vi "dfd_MRate_Calculate Filter Gain.vi"(9 "scale type":T3=enum."Time Domain 1-Norm", 10 "scale by Power of 2?":bool, 11 "multirate filter in":T1={"mMRate_Structure"=enum."CIC", "mMRate_Mode"=0, "mMRate_Factor"=0, "mMRate_FIRParams"={"mMRate_FIR_H"=[], "mMRate_FIR_IsNyquist?"=FALSE, "mMRate_FIR_IsSymmetric?"=FALSE}, "mMRate_CICParams"={"mMRate_CIC_#Stage"=0, "mMRate_CIC_Lag"=0, "mMRate_CIC_Type"=enum."Lowpass"}, "mMRate_Order"=0, "mMRate_Version"="", "mMRate_Comments"="", "mMRate_RationalFactor"={"mMRate_L"=-1, "mMRate_M"=-1}, "mMRate_Fs"=0.0, "mMRate_Quantized?"=FALSE, "mMRate_QFilterGain"=1.0, "mMRate_CoefWl"=16, "mMRate_Scaling"={"mMRate_ScaleByPowerOf2?"=FALSE, "mMRate_ScaleType"=enum."Time Domain 1-Norm"}, "mMRate_InputWl"=0, "mMRate_OutputWl"=0, "mMRate_OutputMode"=enum."Nearest", "mMRate_MultMode"=enum."Truncated", "mMRate_BitPruning"=FALSE, "mMRate_GainWl"=16, "mMRate_OutputFwl"=0, "mMRate_SumIwl"=0, "mMRate_InputIwl "=16, "mMRate_SumWl"=32, "mMRate_CoefIwl"=0} {"mMRate_SumWl" min=1 max=32 step=1; "mMRate_InputIwl" min=1 max=32 step=1; "mMRate_GainWl" min=1 max=32 step=1; "mMRate_OutputWl" min=1 max=32 step=1; "mMRate_InputWl" min=1 max=32 step=1; "mMRate_CoefWl" min=1 max=32 step=1; "mMRate_Mode" items=["Default"=-1, "No Rate Change"=0, "Interpolation"=1, "Decimation"=2, "Interpolated"=3, "Rational"=4]}) -> (1 "sum iwl":i16, 2 "scaled gain":dbl, 3 "dup multirate filter":T1={"mMRate_Structure"=enum."CIC", "mMRate_Mode"=0, "mMRate_Factor"=0, "mMRate_FIRParams"={"mMRate_FIR_H"=[], "mMRate_FIR_IsNyquist?"=FALSE, "mMRate_FIR_IsSymmetric?"=FALSE}, "mMRate_CICParams"={"mMRate_CIC_#Stage"=0, "mMRate_CIC_Lag"=0, "mMRate_CIC_Type"=enum."Lowpass"}, "mMRate_Order"=0, "mMRate_Version"="", "mMRate_Comments"="", "mMRate_RationalFactor"={"mMRate_L"=-1, "mMRate_M"=-1}, "mMRate_Fs"=0.0, "mMRate_Quantized?"=FALSE, "mMRate_QFilterGain"=1.0, "mMRate_CoefWl"=16, "mMRate_Scaling"={"mMRate_ScaleByPowerOf2?"=FALSE, "mMRate_ScaleType"=enum."Time Domain 1-Norm"}, "mMRate_InputWl"=0, "mMRate_OutputWl"=0, "mMRate_OutputMode"=enum."Nearest", "mMRate_MultMode"=enum."Truncated", "mMRate_BitPruning"=FALSE, "mMRate_GainWl"=16, "mMRate_OutputFwl"=0, "mMRate_SumIwl"=0, "mMRate_InputIwl "=16, "mMRate_SumWl"=32, "mMRate_CoefIwl"=0} {"mMRate_SumWl" min=1 max=32 step=1; "mMRate_InputIwl" min=1 max=32 step=1; "mMRate_GainWl" min=1 max=32 step=1; "mMRate_OutputWl" min=1 max=32 step=1; "mMRate_InputWl" min=1 max=32 step=1; "mMRate_CoefWl" min=1 max=32 step=1; "mMRate_Mode" items=["Default"=-1, "No Rate Change"=0, "Interpolation"=1, "Decimation"=2, "Interpolated"=3, "Rational"=4]})   [LabVIEW 2017, in "NI_DigFilter_FXP.lvlib"]
uses:
  <vilib>/addons/Digital Filter Design/NI_DigFilter_FXP.lvlib
  <vilib>/addons/Digital Filter Design/_Objects.llb/DFD Coef Norm Type.ctl
  <vilib>/addons/Digital Filter Design/_Objects.llb/DFD Multirate Filter Obj.ctl
  <vilib>/addons/Digital Filter Design/_Objects.llb/DFD Multirate Mode.ctl
  <vilib>/addons/Digital Filter Design/_Objects.llb/DFD Round-off Mode.ctl
  <vilib>/addons/Digital Filter Design/_Objects.llb/DFD FXP MRate Multiply Mode.ctl
  <vilib>/addons/Digital Filter Design/NI_DigFilterLicensed.lvlib
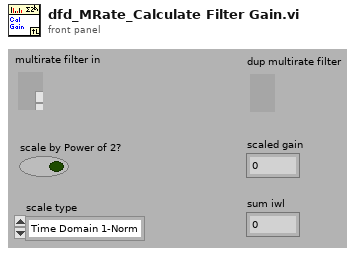
[diagram p1: front panel]
types:
  T1 = typedef "NI_DigFilterLicensed.lvlib/DFD Multirate Filter Obj.ctl" = cluster{"mMRate_Structure":enum16{"CIC", "FIR", "IIR", "Lattice"}, "mMRate_Mode":T2, "mMRate_Factor":i32, "mMRate_FIRParams":cluster{"mMRate_FIR_H":dbl[], "mMRate_FIR_IsNyquist?":bool, "mMRate_FIR_IsSymmetric?":bool}, "mMRate_CICParams":cluster{"mMRate_CIC_#Stage":i32, "mMRate_CIC_Lag":i32, "mMRate_CIC_Type":enum16{"Lowpass", "Highpass"}}, "mMRate_Order":i32, "mMRate_Version":string, "mMRate_Comments":string, "mMRate_RationalFactor":cluster{"mMRate_L":i32, "mMRate_M":i32}, "mMRate_Fs":dbl, "mMRate_Quantized?":bool, "mMRate_QFilterGain":dbl, "mMRate_CoefWl":i16, "mMRate_Scaling":cluster{"mMRate_ScaleByPowerOf2?":bool, "mMRate_ScaleType":T3}, "mMRate_InputWl":i16, "mMRate_OutputWl":i16, "mMRate_OutputMode":T4, "mMRate_MultMode":T5, "mMRate_BitPruning":bool, "mMRate_GainWl":i16, "mMRate_OutputFwl":i16, "mMRate_SumIwl":i16, "mMRate_InputIwl ":i16, "mMRate_SumWl":i16, "mMRate_CoefIwl":i16}
  T2 = typedef "NI_DigFilterLicensed.lvlib/DFD Multirate Mode.ctl" = i16
  T3 = typedef "NI_DigFilterLicensed.lvlib/DFD Coef Norm Type.ctl" = enum16{"No Norm", "Time Domain 1-Norm", "Time Domain 2-Norm", "Time Domain Inf-Norm"}
  T4 = typedef "NI_DigFilterLicensed.lvlib/DFD Round-off Mode.ctl" = enum16{"Nearest", "Truncation"}
  T5 = typedef "NI_DigFilterLicensed.lvlib/DFD FXP MRate Multiply Mode.ctl" = enum16{"Truncated", "Full"}
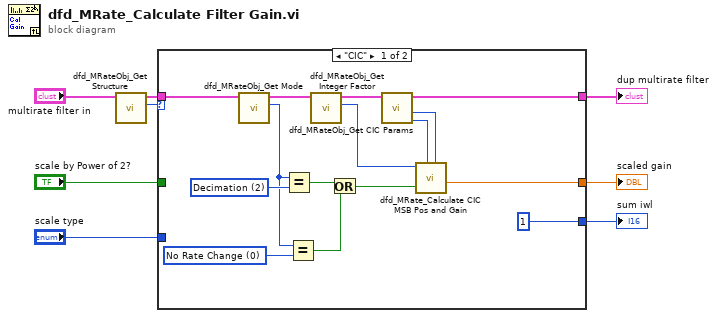
[diagram p0: block diagram]
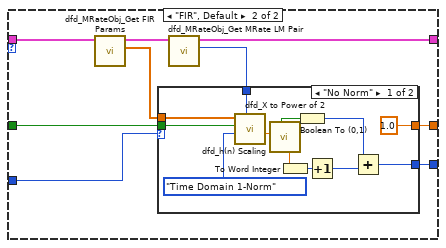
[diagram p2: hidden frame]
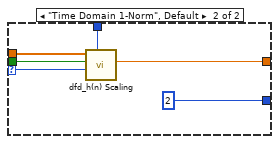
[diagram p3: hidden frame]
diagram:
  n1 = call <vilib>:"dfd_MRateObj_Get Structure.vi"("multirate filter in"="multirate filter in") -> ("structure"=w6:enum16{"CIC", "FIR", "IIR", "Lattice"}, "dup multirate filter"=w5:T1)  [unwired: 9 out]
  n2 = case shown="\"CIC\"" w6 {
    tunnel: "scale type" -> [_ w25]
    tunnel: [w14 w30] -> w8
    tunnel: w5 -> [w22 w32]
    tunnel: [w17 w27] -> w4
    tunnel: "scale by Power of 2?" -> [_ w31]
    tunnel: [i16 1 w24] -> w1
    frame "CIC" {
      w11 = T2 0 items=["Default"=-1, "No Rate Change"=0, "Interpolation"=1, "Decimation"=2, "Interpolated"=3, "Rational"=4] ("y")
      w23 = T2 2 items=["Default"=-1, "No Rate Change"=0, "Interpolation"=1, "Decimation"=2, "Interpolated"=3, "Rational"=4] ("y")
      n3 = call <vilib>:"dfd_MRateObj_Get Mode.vi"("multirate filter in"=w22) -> ("mode"=w12:T2, "dup multirate filter"=w19:T1)  [unwired: 9 out]
      n4 = Equal?(x=w12, y=w23) -> (x = y?=w13:bool)
      n5 = Equal?(x=w12, y=w11) -> (x = y?=w10:bool)
      n6 = call <vilib>:"dfd_MRateObj_Get Integer Factor.vi"("multirate filter in"=w19) -> ("factor"=w15:i32, "dup multirate filter"=w18:T1)  [unwired: 9 out]
      n7 = Or(x=w13, y=w10) -> (x .or. y?=w9:bool)
      n8 = call <vilib>:"dfd_MRateObj_Get CIC Params.vi"("multirate filter in"=w18) -> ("lag"=w21:i32, "# stages"=w20:i32, "dup multirate filter"=w17:T1)  [unwired: 8 out]
      n9 = call <vilib>:"dfd_MRate_Calculate CIC MSB Pos and Gain.vi"("#stage"=w20, "Decimation? (T)"=w9, "lag"=w21, "factor"=w15) -> ("filter gain"=w14:dbl)  [unwired: 7 out]
    }
    frame "FIR", Default {
      n10 = call <vilib>:"dfd_MRateObj_Get FIR Params.vi"("multirate filter in"=w32) -> ("h(n)"=w29:dbl[], "dup multirate filter"=w28:T1)  [unwired: 9 out]
      n11 = call <vilib>:"dfd_MRateObj_Get MRate LM Pair.vi"("multirate filter in"=w28) -> ("L"=w26:i32, "dup multirate filter"=w27:T1)  [unwired: 1 in, 8 out]
      n12 = case shown="\"No Norm\"" w25 {
        selector: w25 -> [_ w47]
        tunnel: w31 -> [w42 w50]
        tunnel: [1.0 ("scale value") w46] -> w30
        tunnel: w29 -> [w44 w49]
        tunnel: w26 -> [w43 w48]
        tunnel: [w35 i16 2] -> w24
        frame "No Norm" {
          n13 = call <vilib>:"dfd_h(n) Scaling.vi"("L"=w43, "scale type"=DFD_Coef_Norm_Type."Time Domain 1-Norm", "scale by Power of 2?"=w42, "h(n)"=w44) -> ("norm value"=w39:dbl)  [unwired: 7 out]
          n14 = call <vilib>:"dfd_X to Power of 2.vi"("x"=w39) -> ("n"=w38:dbl, "is 2^n?"=w34:bool)  [unwired: 9 out]
          n15 = To Word Integer(number=w38) -> (16bit integer=w37:i16)
          n16 = Boolean To (0,1)(Boolean=w34) -> (0, 1=w33:i16)
          n17 = Increment(x=w37) -> (x+1=w36:i16)
          n18 = Add(x=w33, y=w36) -> (x+y=w35:i16)
        }
        frame "Time Domain 1-Norm", Default {
          n19 = call <vilib>:"dfd_h(n) Scaling.vi"("L"=w48, "scale type"=w47, "scale by Power of 2?"=w50, "h(n)"=w49) -> ("scale value"=w46:dbl)  [unwired: 7 out]
        }
      }
    }
  }
  "scaled gain" <- w8
  "dup multirate filter" <- w4
  "sum iwl" <- w1
